vi "WriteString.vi"(8 "To apppend":string, 11 "Original string":string) -> (3 "Appended string":string)   [LabVIEW 2017, in "LeapMotion.lvlib"]
uses:
  LeapMotion.lvlib
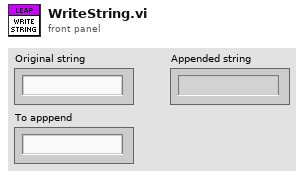
[diagram p1: front panel]
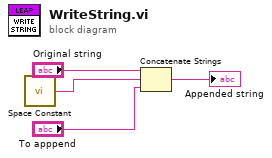
[diagram p0: block diagram]
diagram:
  n1 = call <vilib>:"Space Constant.vi"() -> ("String"=w2:string)
  n2 = Concatenate Strings("Original string", w2, "To apppend") -> (→"Appended string":string)
